vi "OAT Even Time or Speed Segment (XY, 2D Array).vi"(0 "XY signals":cluster{"X":dbl[], "Y":dbl[]}[][](array[cluster]) {"X" format="%.2f"; "Y" format="%.2f"}, 1 "x-axis selection":u16(ring)=2 items=["Time", "Revolution", "RPM"], 2 "reset? (F)":bool, 3 "phase input? (F)":bool, 5 "speed profile":T4 {"speed [RPM]" format="%.2f"; "time [s]" format="%.2f"}, 7 "position info":T2, 9 "pulse/revolution (1)":i32=1, 11 "error in (no error)":errorcluster, 12 "segment settings":cluster{"start":dbl, "end":dbl, "step size":dbl} {"step size" format="%.2f"; "end" min=0.0 format="%.2f"; "start" min=0.0 format="%.2f"}, 13 "view info":T1={"dB on? (F)"=FALSE, "unwrap phase? (T)"=TRUE, "unit in degree? (T)"=TRUE}) -> (4 "XY signals out":cluster{"X":dbl[], "Y":dbl[]}[][](array[cluster]) {"X" format="%.2f"; "Y" format="%.2f"}, 8 "position info out":T2, 10 "end reached?":bool, 14 "actual segment settings":T3 {"actual step size" format="%.2f"; "actual end" min=0.0 format="%.2f"; "actual start" min=0.0 format="%.2f"}, 15 "error out":errorcluster)   [LabVIEW 2017, in "SoundVib_OAUtility.lvlib"]
doc: "Divides an input signal into even-time segments or even-speed intervals. The input signal of this VI can be an even-angle signal or an XY signal. When you use this VI to divide an XY signal, the XY signal can be only the output of the OAT Order Magnitude and Phase VI or OAT Overall Level Plot VI. Wire data to the <B>even-angle signal</B> input to determine the polymorphic instance to use or manually select the instance."
uses:
  <vilib>/addons/Sound and Vibration/Order Analysis/Utility/SoundVib_OAUtility.lvlib
  <vilib>/addons/Sound and Vibration/Order Analysis/Tach Process/SubVIs/speed profile.ctl
  <vilib>/addons/Sound and Vibration/Order Analysis/Misc/OAT Position Info.ctl
  <vilib>/addons/Sound and Vibration/Order Analysis/Tach Process/SoundVib_TachProcess.lvlib
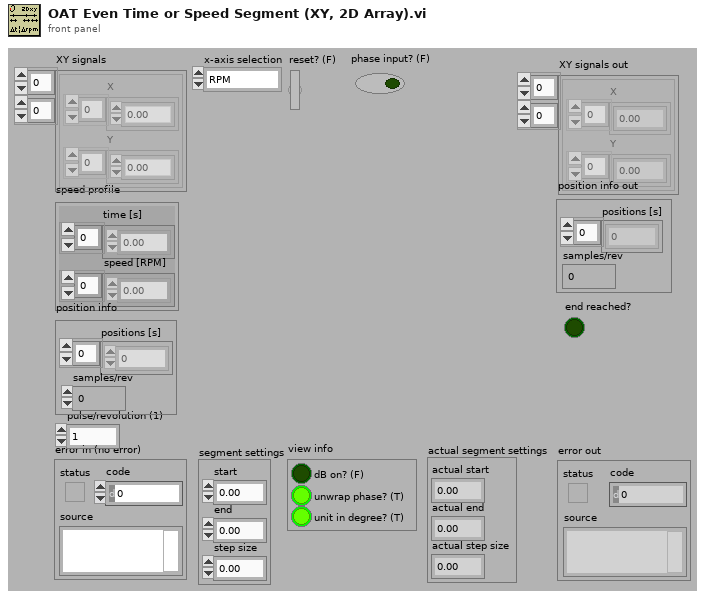
[diagram p1: front panel]
types:
  T1 = cluster{"dB on? (F)":bool, "unwrap phase? (T)":bool, "unit in degree? (T)":bool}
  T2 = typedef "OAT Position Info.ctl" = cluster{"positions [s]":dbl[], "samples/rev":dbl}
  T3 = cluster{"actual start":dbl, "actual end":dbl, "actual step size":dbl}
  T4 = typedef "SoundVib_TachProcess.lvlib/speed profile.ctl" = cluster{"time [s]":dbl[], "speed [RPM]":dbl[]}
  T5 = cluster{"last rev":dbl, "rev indice":dbl[], "time indice":dbl[], "RPM indice":dbl[]}
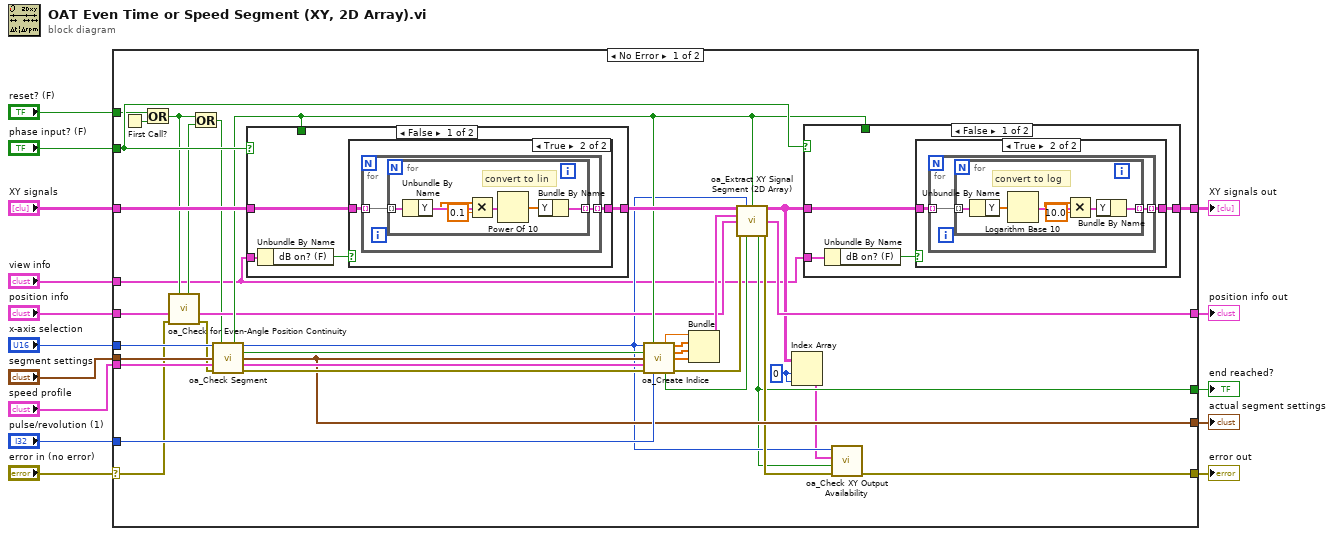
[diagram p0: block diagram]
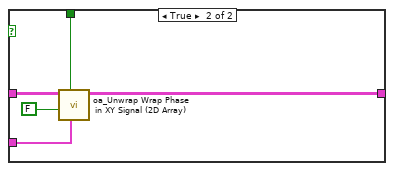
[diagram p3: hidden frame]
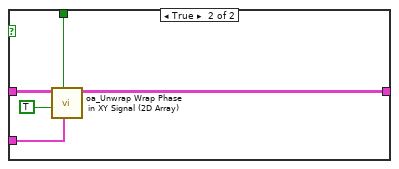
[diagram p5: hidden frame]
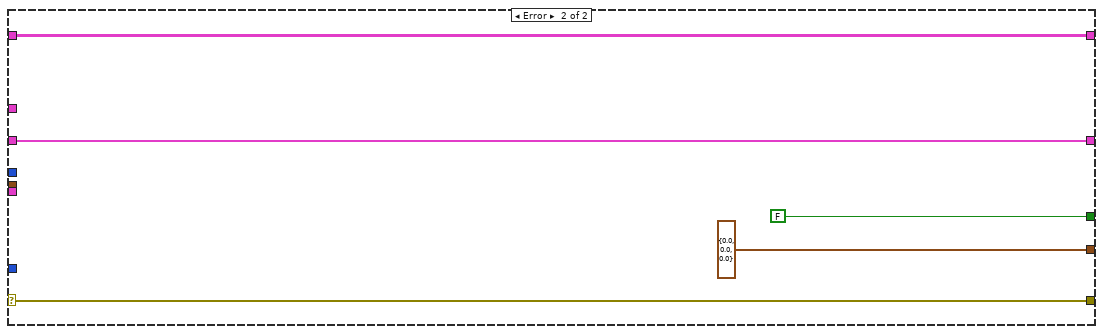
[diagram p6: hidden frame]
diagram:
  n1 = case shown="No Error" "error in (no error)" {
    selector: "error in (no error)" -> [w27 w98]
    tunnel: [w22 w98] -> w1
    tunnel: "reset? (F)" -> [w33 _]
    tunnel: "x-axis selection" -> [w46 _]
    tunnel: "segment settings" -> [w45 _]
    tunnel: "speed profile" -> [w44 _]
    tunnel: [w42 cluster{"start":dbl, "end":dbl, "step":dbl} {"start"=0.0, "end"=0.0, "step"=0.0} ("steps output")] -> w2
    tunnel: "pulse/revolution (1)" -> [w43 _]
    tunnel: "XY signals" -> [w37 w96]
    tunnel: [w20 FALSE ("finish?")] -> w4
    tunnel: "position info" -> [w40 w95]
    tunnel: [w35 w96] -> w5
    tunnel: [w38 w95] -> w3
    tunnel: "phase input? (F)" -> [w34 _]
    tunnel: "view info" -> [w16 _]
    frame No Error {
      w17 = 0 ("index (row)")
      n2 = First Call?() -> (First Call?: T/F=w32:bool)
      n3 = Or(x=w33, y=w32) -> (x .or. y?=w25:bool)
      n4 = call <vilib>:"oa_Check for Even-Angle Position Continuity.vi"("reset in"=w25, "error in (no error)"=w27, "even-angle position info"=w40) -> ("error out"=w28:errorcluster, "even-angle position info dup"=w29:T2, "position not continuous"=w24:bool)  [unwired: 6 in]
      n5 = Or(x=w25, y=w24) -> (x .or. y?=w26:bool)
      n6 = call <vilib>:"oa_Check Segment.vi"("X axis selection"=w46, "reset?(F)"=w26, "segment position"=w45, "speed profile"=w44, "error in (no error)"=w28) -> ("reset out"=w30:bool, "X axis selection"=w21:u16, "step found?"=w51:bool, "segment position out"=w42:cluster{"start":dbl, "end":dbl, "step size":dbl}, "dul speed profile"=w52:T4, "error out"=w53:errorcluster)  [unwired: 5 in]
      n7 = case shown="False" w34 {
        tunnel: w37 -> [w75 w93]
        tunnel: [w74 w92] -> w36
        tunnel: w16 -> [w77 w91]
        tunnel: w30 -> [_ w90]
        frame False {
          n8 = Unbundle By Name(w77) -> ("dB on? (F)"=w76:bool)
          n9 = case shown="True" w76 {
            tunnel: w75 -> [w78 w80]
            tunnel: [w78 w79] -> w74
            frame False {
            }
            frame True {
              n10 = for {
                tunnel: w80 -> [w82] mode=indexing
                tunnel: [w81] -> w79 mode=indexing
                n11 = for {
                  tunnel: w82 -> [w87] mode=indexing
                  tunnel: [w86] -> w81 mode=indexing
                  # "convert to lin"
                  n12 = Unbundle By Name(w87) -> ("Y"=w84:dbl[])
                  n13 = Multiply(x=w84, y=0.1) -> (x*y=w83:dbl[])
                  n14 = Power Of 10(x=w83) -> (10^x=w88:dbl[])
                  n15 = Bundle By Name(cluster=w87, "Y"=w88) -> (w86:cluster{"X":dbl[], "Y":dbl[]})
                }
              }
            }
          }
        }
        frame True {
          n16 = call <vilib>:"oa_Unwrap Wrap Phase in XY Signal (2D Array).vi"("view"=w91, "reset? (F)"=w90, "Unwrap?"=TRUE, "XY signals"=w93) -> ("XY signals out"=w92:cluster{"X":dbl[], "Y":dbl[]}[][])  [unwired: 7 in]
        }
      }
      n17 = call <vilib>:"oa_Create Indice.vi"("X axis selection"=w21, "reset?(F)"=w30, "step found?(F)"=w51, "steps input"=w42, "speed profile"=w52, "error in (no error)"=w53, "pulse/revolution (1)"=w43) -> ("last rev"=w47:dbl, "rev indice"=w48:dbl[], "time indice"=w49:dbl[], "RPM indice"=w50:dbl[], "reach end?"=w31:bool, "error out"=w39:errorcluster)  [unwired: 2 in, 1 out]
      n18 = Bundle("last rev"=w47, "rev indice"=w48, "time indice"=w49, "RPM indice"=w50) -> (w41:T5)  [unwired: 1 in]
      n19 = call <vilib>:"oa_Extract XY Signal Segment (2D Array).vi"("XY signals"=w36, "X axis selection"=w21, "reset? (F)"=w30, "trigger indices"=w41, "position info in"=w29, "error in (no error)"=w39, "indices end?"=w31) -> ("XY signals out"=w19:cluster{"X":dbl[], "Y":dbl[]}[][], "position info out"=w38:T2, "reached end?"=w20:bool, "error out"=w23:errorcluster)  [unwired: 5 in]
      n20 = Index Array(array=w19, index (row)=w17, index (col)=w17) -> (element=w18:cluster{"X":dbl[], "Y":dbl[]})
      n21 = case shown="False" w34 {
        tunnel: w19 -> [w55 w73]
        tunnel: [w54 w72] -> w35
        tunnel: w30 -> [_ w70]
        tunnel: w16 -> [w56 w69]
        frame False {
          n22 = Unbundle By Name(w56) -> ("dB on? (F)"=w57:bool)
          n23 = case shown="True" w57 {
            tunnel: w55 -> [w58 w60]
            tunnel: [w58 w59] -> w54
            frame False {
            }
            frame True {
              n24 = for {
                tunnel: w60 -> [w62] mode=indexing
                tunnel: [w61] -> w59 mode=indexing
                n25 = for {
                  tunnel: w62 -> [w67] mode=indexing
                  tunnel: [w66] -> w61 mode=indexing
                  # "convert to log"
                  n26 = Unbundle By Name(w67) -> ("Y"=w68:dbl[])
                  n27 = Logarithm Base 10(1:w68) -> (0:w64:dbl[])
                  n28 = Multiply(x=w64, y=10.0) -> (x*y=w63:dbl[])
                  n29 = Bundle By Name(cluster=w67, "Y"=w63) -> (w66:cluster{"X":dbl[], "Y":dbl[]})
                }
              }
            }
          }
        }
        frame True {
          n30 = call <vilib>:"oa_Unwrap Wrap Phase in XY Signal (2D Array).vi"("view"=w69, "reset? (F)"=w70, "Unwrap?"=FALSE, "XY signals"=w73) -> ("XY signals out"=w72:cluster{"X":dbl[], "Y":dbl[]}[][])  [unwired: 7 in]
        }
      }
      n31 = call <vilib>:"oa_Check XY Output Availability.vi"("error in (no error)"=w23, "reached end?"=w20, "XY signal"=w18, "x-axis selection"=w21) -> ("error out"=w22:errorcluster)  [unwired: 7 in]
    }
    frame Error {
    }
  }
  "error out" <- w1
  "end reached?" <- w4
  "actual segment settings" <- w2
  "XY signals out" <- w5
  "position info out" <- w3
